vi "Generate Signal.vi"(4 "Error In":errorcluster, 6 "Signal Data":variant, 7 "Notifier Name":string) -> (0 "Error Out":errorcluster)   [LabVIEW 2015, in "not_Generic Named Notifier.lvlib"]
uses:
  not_Generic Named Notifier.lvlib
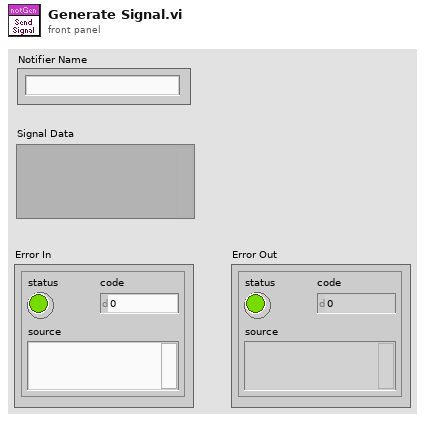
[diagram p1: front panel]
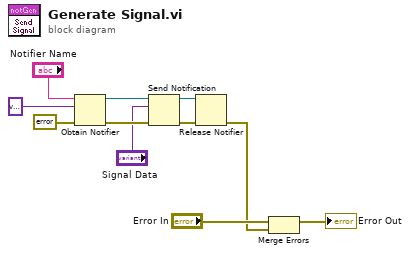
[diagram p0: block diagram]
diagram:
  n1 = Obtain Notifier(name (unnamed)="Notifier Name", notification data type=variant ("element data type"), error in (no error)=errorcluster {"status"=FALSE, "code"=0, "source"=""}) -> (notifier out=w10:refnum<notifier>, error out=w11:errorcluster)  [unwired: 1 in, 1 out]
  n2 = Send Notification(notification="Signal Data", notifier=w10, error in (no error)=w11) -> (notifier out=w9:refnum<notifier>, error out=w8:errorcluster)
  n3 = Release Notifier(notifier=w9, error in (no error)=w8) -> (error out=w2:errorcluster)  [unwired: 1 in, 2 out]
  n4 = Merge Errors("Error In", w2) -> (→"Error Out":errorcluster)
